vi "JSON-DBUpdate.vi"(0 "Table":string="Inventory", 2 "Column Number":string="Inventory", 5 "SQL Statement":string, 11 "error in":errorcluster, 12 "Data":string="ReplyWithAddQuery") -> (4 "Output JSON Object":string, 15 "error out":errorcluster)   [LabVIEW 2013]
uses:
  ftw-dataflow/Actor/src/Utility/FTW-Actor-Configuration.ctl
  ftw-dataflow/Actor/src/FTW-Actor.lvlib
panel:
  in  "Update All":bool
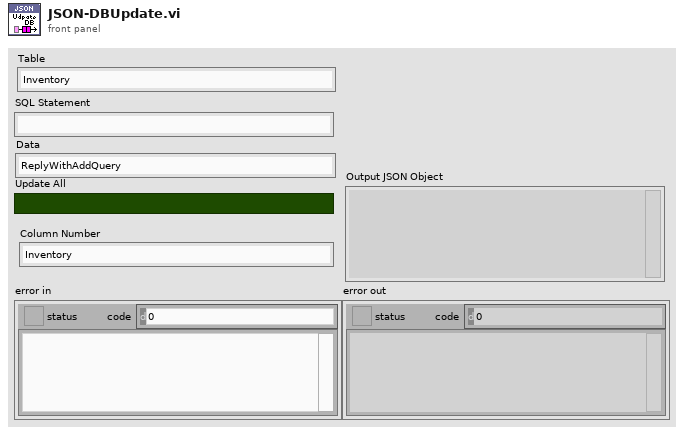
[diagram p1: front panel]
types:
  T1 = typedef "FTW-Actor.lvlib/FTW-Actor-Configuration.ctl" = string
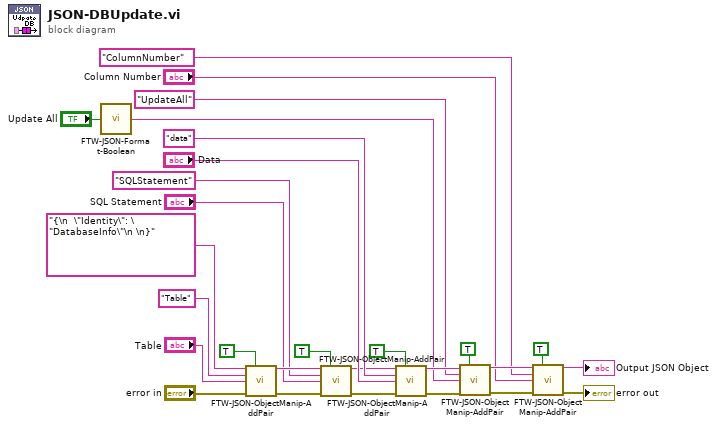
[diagram p0: block diagram]
diagram:
  n1 = call "FTW-JSON-Format-Boolean.vi"("LabVIEW Boolean"="Update All") -> ("JSON Boolean"=w2:string)
  n2 = call "FTW-JSON-ObjectManip-AddPair.vi"("Input JSON Object"=T1 "{\n  \"Identity\": \"DatabaseInfo\"\n \n}" ("FTW Actor Instance Configuration 2"), "Escape Value to String?"=TRUE, "Key"="Table", "Value"="Table", "error in"="error in") -> ("Output JSON Object"=w24:string, "error out"=w15:errorcluster)  [unwired: 9 in]
  n3 = call "FTW-JSON-ObjectManip-AddPair.vi"("Input JSON Object"=w24, "Escape Value to String?"=TRUE, "Key"="SQLStatement", "Value"="SQL Statement", "error in"=w15) -> ("Output JSON Object"=w26:string, "error out"=w14:errorcluster)  [unwired: 9 in]
  n4 = call "FTW-JSON-ObjectManip-AddPair.vi"("Input JSON Object"=w26, "Escape Value to String?"=TRUE, "Key"="data", "Value"="Data", "error in"=w14) -> ("Output JSON Object"=w13:string, "error out"=w12:errorcluster)  [unwired: 9 in]
  n5 = call "FTW-JSON-ObjectManip-AddPair.vi"("Input JSON Object"=w13, "Escape Value to String?"=TRUE, "Key"="UpdateAll", "Value"=w2, "error in"=w12) -> ("Output JSON Object"=w8:string, "error out"=w7:errorcluster)  [unwired: 9 in]
  n6 = call "FTW-JSON-ObjectManip-AddPair.vi"("Input JSON Object"=w8, "Escape Value to String?"=TRUE, "Key"="ColumnNumber", "Value"="Column Number", "error in"=w7) -> ("Output JSON Object"=→"Output JSON Object":string, "error out"=→"error out":errorcluster)  [unwired: 9 in]
